vi "updateActuatorSetpoint.vi"(8 "error in (no error)":errorcluster, 11 "Model in":refnum<class "Model.lvclass">) -> (0 "error out":errorcluster, 3 "Model out":refnum<class "Model.lvclass">)   [LabVIEW 2015, in "Model.lvclass"]
uses:
  Model.lvclass
  Model.lvclass/Model.ctl
  Actuator/IActuator/IActuator.lvclass
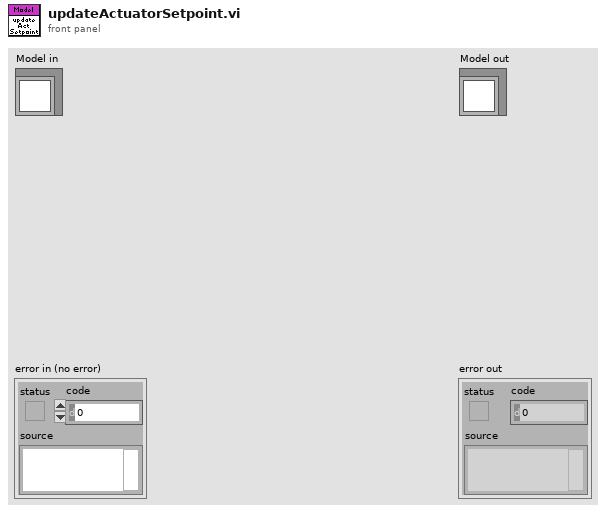
[diagram p1: front panel]
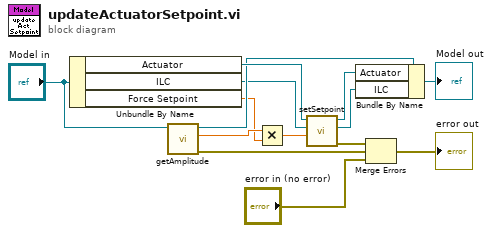
[diagram p0: block diagram]
diagram:
  n1 = Unbundle By Name("Model in") -> ("Actuator"=w14:refnum<class "IActuator.lvclass">, "ILC"=w5:refnum<class "ILC.lvclass">, "Force Setpoint"=w1:dbl[unit])
  n2 = call "getAmplitude.vi"("Model in"="Model in") -> ("error out"=w6:errorcluster, "Result"=w3:dbl, "Model out"=w12:refnum<class "Model.lvclass">)  [unwired: 8 in]
  n3 = Multiply(x=w3, y=w1) -> (x*y=w2:dbl[unit])
  n4 = call-dynamic "setSetpoint.vi"("Force Setpoint"=w2, "ILC in"=w5, "IActuator in"=w14) -> ("error out"=w7:errorcluster, "ILC out"=w4:refnum<class "ILC.lvclass">, "IActuator out"=w10:refnum<class "IActuator.lvclass">)  [unwired: 6 in]
  n5 = Bundle By Name(cluster=w12, "Actuator"=w10, "ILC"=w4) -> (→"Model out":refnum<class "Model.lvclass">)
  n6 = Merge Errors(w7, w6, "error in (no error)") -> (→"error out":errorcluster)
